vi "ValidateResults.vi"(8 "error in (no error)":errorcluster, 11 "Prime_Sieve in":refnum<class "Prime_Sieve.lvclass">) -> (0 "error out":errorcluster, 2 "Valid Results?":bool, 3 "Prime_Sieve out":refnum<class "Prime_Sieve.lvclass">)   [LabVIEW 2020, in "Prime_Sieve.lvclass"]
uses:
  Prime_Sieve.lvclass
  Prime_Sieve.lvclass/Prime_Sieve.ctl
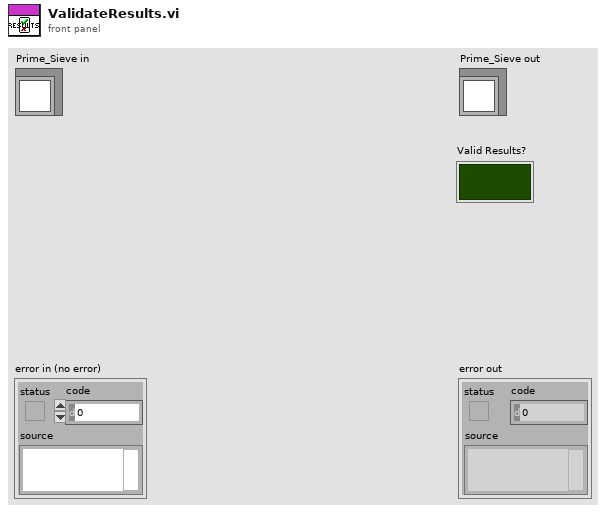
[diagram p1: front panel]
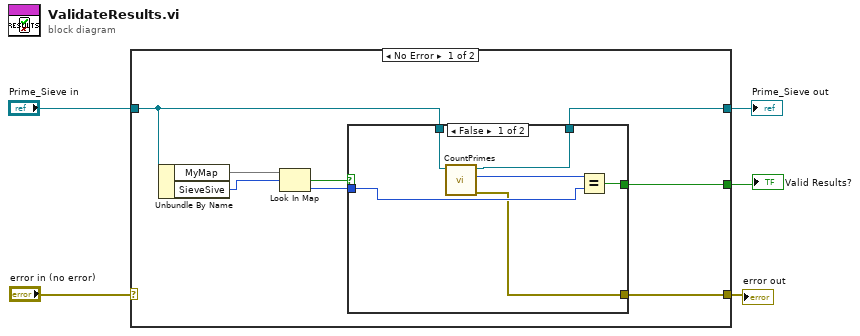
[diagram p0: block diagram]
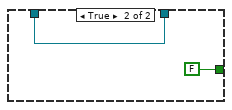
[diagram p2: hidden frame]
diagram:
  n1 = case shown="No Error" "error in (no error)" {
    selector: "error in (no error)" -> [_ w23]
    tunnel: [w6 w23] -> w4
    tunnel: [w9 w22] -> w2
    tunnel: "Prime_Sieve in" -> [w8 w22]
    tunnel: [w10 _] -> w1
    frame No Error {
      n2 = Unbundle By Name(w8) -> ("MyMap"=w13:map{i64, i32}, "SieveSive"=w12:i64)
      n3 = Look In Map(map=w13, key=w12) -> (key not found?=w11:bool, value=w7:i32)  [unwired: 1 in]
      n4 = case shown="False" w11 {
        tunnel: [w17 FALSE] -> w10
        tunnel: w8 -> [w19 w20]
        tunnel: [w18 w20] -> w9
        tunnel: w7 -> [w15 _]
        tunnel: [w14 _] -> w6
        frame False {
          n5 = call "CountPrimes.vi"("Prime_Sieve in"=w19) -> ("error out"=w14:errorcluster, "Count"=w16:i32, "Prime_Sieve out"=w18:refnum<class "Prime_Sieve.lvclass">)  [unwired: 8 in]
          n6 = Equal?(x=w16, y=w15) -> (x = y?=w17:bool)
        }
        frame True {
        }
      }
    }
    frame Error {
    }
  }
  "error out" <- w4
  "Prime_Sieve out" <- w2
  "Valid Results?" <- w1
